vi "K to F(2D dbl).vi"(1 "K":dbl[][](array[numeric])) -> (0 "F":dbl[][](array[numeric]))   [LabVIEW 2012, in "Temp Converter.lvlib"]
doc: "<B>输入端子C</B>: 输入开氏温度\n<B>输出端子C</B>: 输出华氏温度。\n\n公式：K-->C-->F\n创建者：CSXCS_366"
uses:
  Temp Converter.lvlib
  KtoC/K to C (2D dbl).vi
  CtoF/C to F (2D dbl).vi
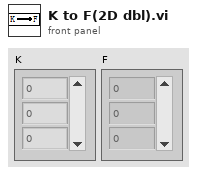
[diagram p1: front panel]
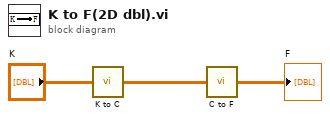
[diagram p0: block diagram]
diagram:
  n1 = call-poly "K to C.vi"("K"="K") -> ("C"=w2:dbl[][])
  n2 = call-poly "C to F.vi"("C"=w2) -> ("F"=→"F":dbl[][])
